vi "encoder2_test_v1.vi"() -> ()   [LabVIEW 2014]
uses:
  <vilib>/rvi/FXPMathLib/FxpSinAndCos/subVIs/nifxpmath_SinAndCos_SimConfig.ctl
  <vilib>/rvi/Emulation/niFpgaGetClockAttributes.vi
  <vilib>/rvi/Emulation/niFpgaSctlEmulationGetInTimedLoop.vi
  <vilib>/rvi/Emulation/niFpgaEmulationReportErrorSimple.vi
  <vilib>/rvi/eio/common/nirviEmuTemplateMethod_errors.vi
  <vilib>/rvi/Emulation/niFpgaProcessEmulError.vi
  <vilib>/rvi/Emulation/niFpgaCriticalErrorInLSC.vi
  <vilib>/rvi/interface/RandomDataEmulation/nirviRandomDataMultiElementFPGAFIFO.vi
  <instcachedir>/0/nirviRandomDataMultiElementFPGAFIFO_AD0CFC12EF974623A9C2E4184BC062B2.lvgen/nirviRandomDataMultiElementFPGAFIFO_AD0CFC12EF974623A9C2E4184BC062B2_028.vi
  <vilib>/rvi/interface/RandomDataEmulation/niFpgaRandomDataHandleErrors.vi
  <vilib>/rvi/FXPMathLib/FxpSinAndCos/simVIs/DllFxpSinAndCosTemp_sub.vi
  <vilib>/eio/EIONode/EIONode.xnode
  <vilib>/rvi/FXPMathLib/FxpMul/XNode/nifxpmath_Multiplier.xnode
  <vilib>/rvi/DataTransferAndStorage/Container/XNode/niFpgaContainer.xnode
  <vilib>/rvi/interface/RandomDataEmulation/nirviRandomDataFpgaMultiElementTemplate.vi
  <vilib>/rvi/FXPMathLib/FxpSinAndCos/XNode/nifxpmath_SinAndCos.xnode
  <vilib>/rvi/FXPMathLib/FxpSub/XNode/nifxpmath_Sub.xnode
  <vilib>/rvi/FXPMathLib/sim/FxpSim.dll
panel:
  in  "Tc_Mavg_mot (uSec)":i32 caption="D_d_M_avg_Tc (uSec)"
  out "omega_mot (M_avg)":fxp<+/-,40,19>
  out "D_d_mot (M_avg)":fxp<+/-,40,19>
  out "omega_mag 2":fxp<+/-,36,13>
  out "D_d_mag 2":fxp<+/-,36,16>
  in  "Tc_Mavg_mag  (uSec)":i32 caption="D_d_M_avg_Tc (uSec)"
  out "D_d_mag (M_avg)":fxp<+/-,40,19>
  out "omega_mag (M_avg)":fxp<+/-,40,19>
  in  "Velocity Est. (mag)":i16(ring) items=["T method", "Mavg method"]
  out "rad (NrTheta)":fxp<+/-,40,20>
  out "D (mm)":fxp<+/-,32,7>
  out "Dr_ramp2":fxp<+/-,64,21>
  out "Ts (s)":fxp<+/-,32,6>
  in  "Dr_ramp (mm)":fxp<+/-,33,7>
  out "Dr_ramp":fxp<+/-,64,21>
  in  "Vr (mm/s)":fxp<+/-,33,7>
  out "omega (rad/s)":fxp<+/-,36,13>
  in  "Encoder":i16(ring) items=["Motor", "Magnetic"]
  in  "Dr_step":fxp<+/-,33,7>
  out "Dr":fxp<+/-,33,10>
  in  "Command type":i16(ring) items=["Step", "Sine", "Ramp", "Ramp2"]
  out "Fmr_P":fxp<+/-,30,15>
  in  "Kp":fxp<+/-,27,14>
  out "D_error":fxp<+/-,36,11>
  out "Dr_sin_d":fxp<+/-,51,12>
  out "Sin omega":fxp<+,20,4>
  out "Dr_sin":fxp<+/-,33,10>
  in  "Sin Mag.":fxp<+/-,32,7>
  in  "Sine frequency (Hz)":fxp<+,16,5>=2.0
  out "Time now (s)":fxp<+,52,14>
  out "va":fxp<+/-,36,7>
  out "vb":fxp<+/-,37,8>
  out "vd_F":fxp<+/-,20,5>
  out "vq_F":fxp<+/-,20,5> format="%.57g"
  in  "Stop Motor":bool
  in  "Ini coe.":bool
  out "D_d_mag":fxp<+/-,36,13>
  out "omega_mag":fxp<+/-,36,13>
  out "D_mag":fxp<+/-,32,7>
  in  "Mag. factor":fxp<+/-,20,2>
  out "mt_mag.":u32
  out "D_d_mot":fxp<+/-,36,13>
  in  "Belt_screw":fxp<+/-,7,7>
  in  "Belt_motor":fxp<+/-,6,6>
  out "D_mot":fxp<+/-,32,7>
  out "rad_mag.":fxp<+/-,40,20>
  out "rad_mot":fxp<+/-,40,20>
  out "mt":u32
  out "omega_mot":fxp<+/-,36,13>
  in  "mt0":u32
  out "Mag. Encoder Position":i32
  in  "Encoder Reset":bool
  out "Encoder Position":i32
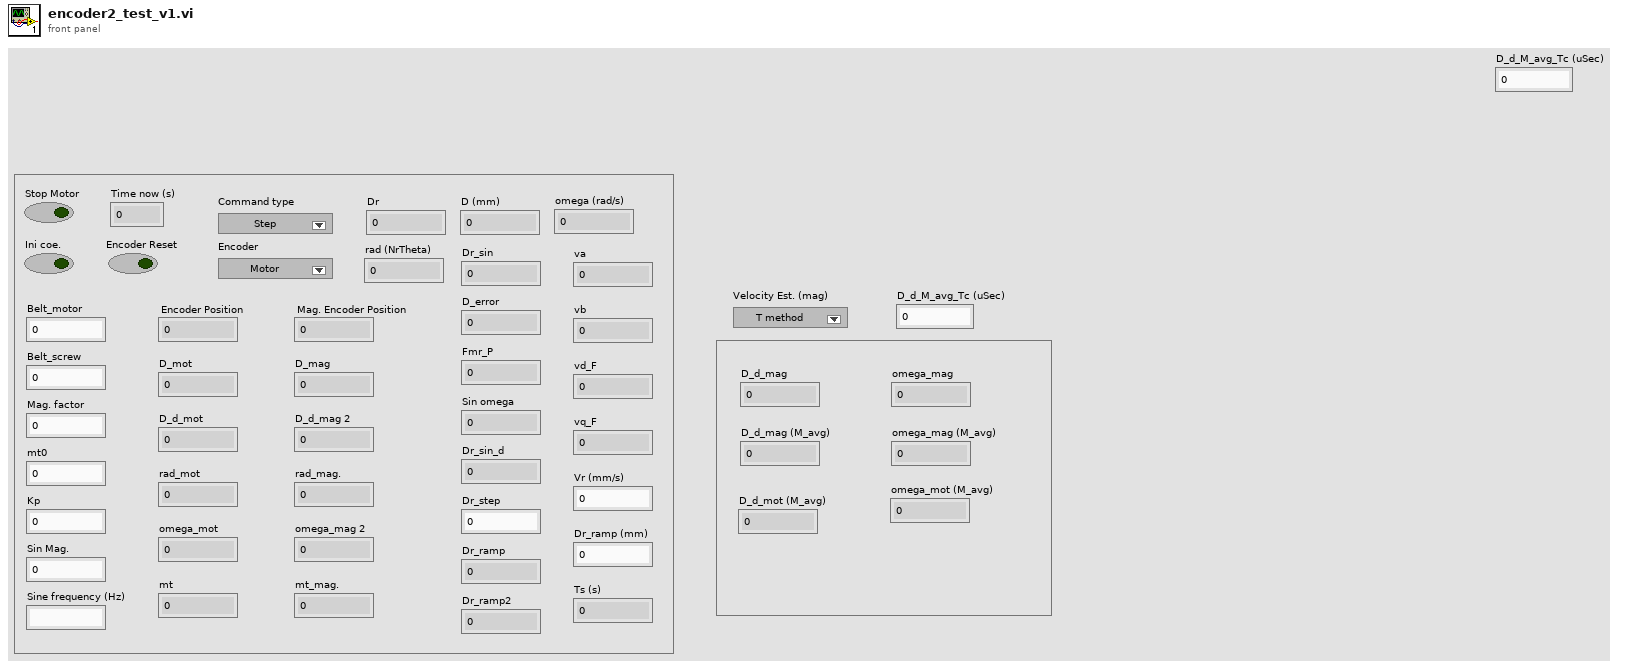
[diagram p1: front panel]
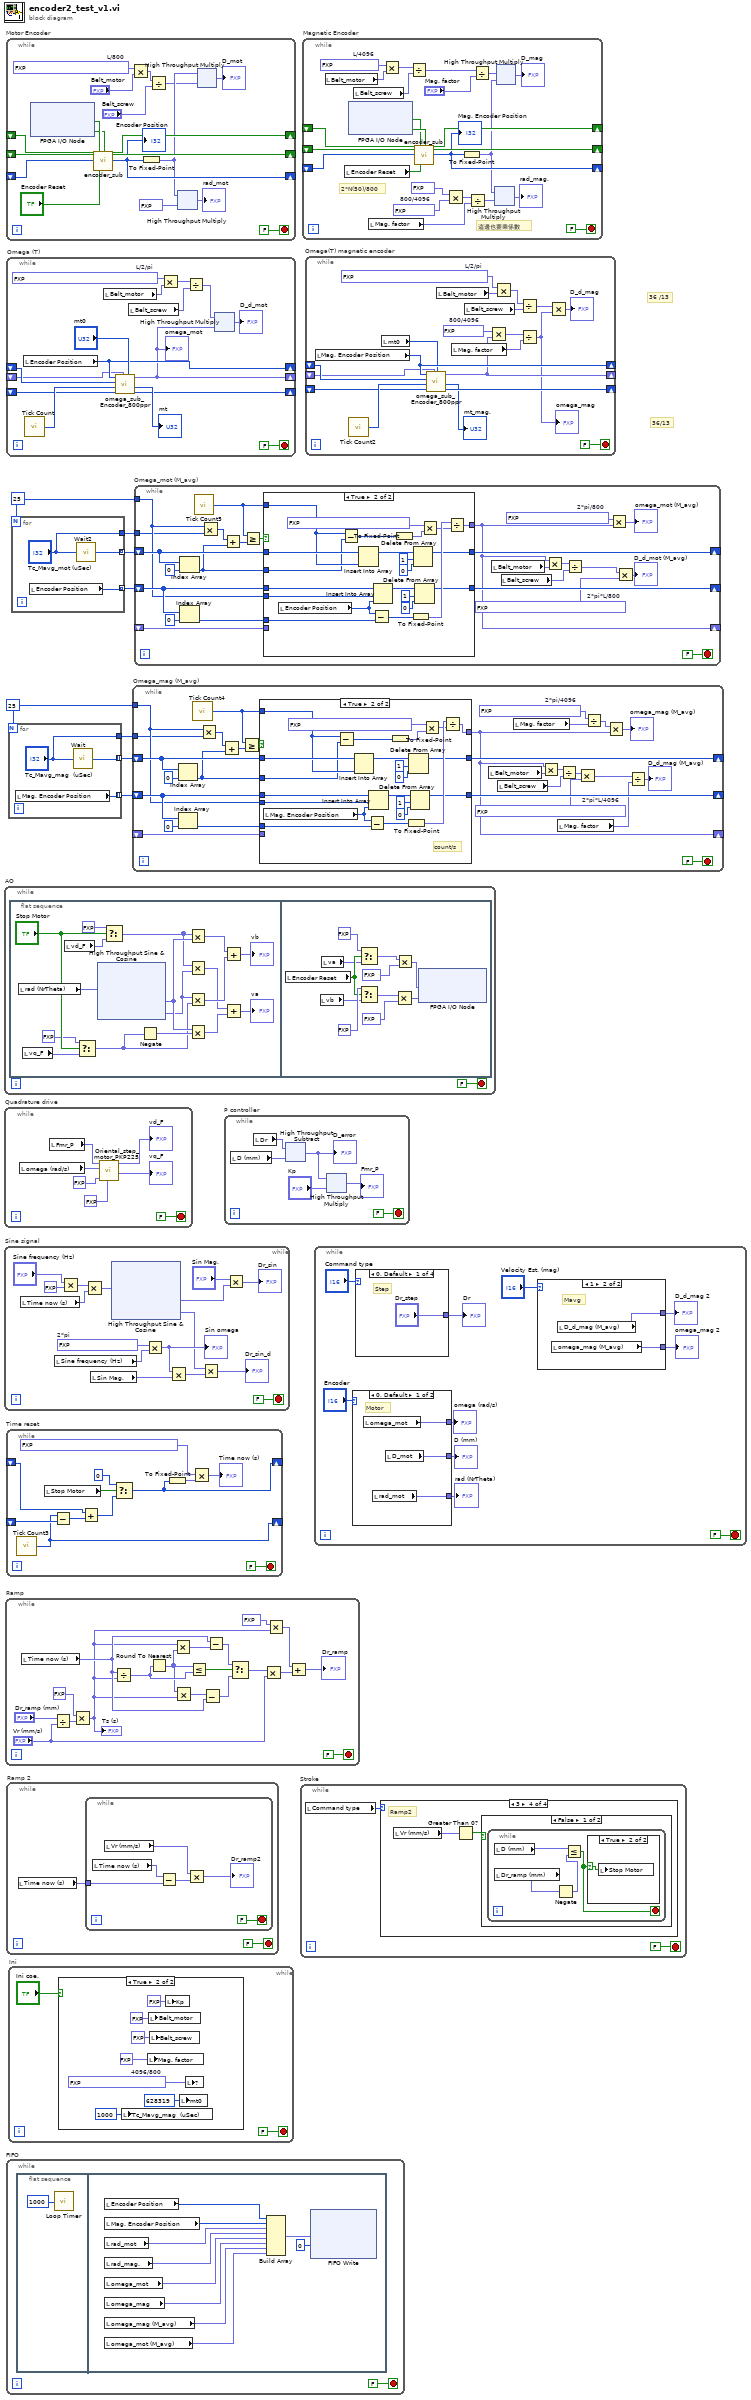
[diagram p0: block diagram]
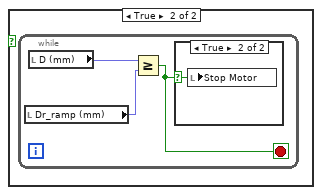
[diagram p8: hidden frame]
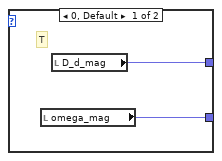
[diagram p10: hidden frame]
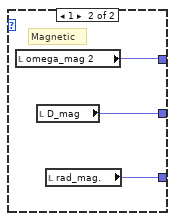
[diagram p11: hidden frame]
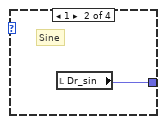
[diagram p12: hidden frame]
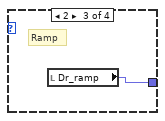
[diagram p13: hidden frame]
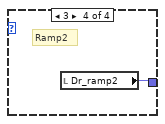
[diagram p14: hidden frame]
diagram:
  w4 = 25
  w8 = 25
  # "36/13"
  # "36 /13"
  n1 = while "AO" {
    stop <- FALSE stop-if-true
    n2 = flat-sequence {
      frame #0 {
        n3 = local read "rad (NrTheta)"() -> (w26:fxp<+/-,40,20>)
        n4 = local read "vq_F"() -> (w22:fxp<+/-,20,5>)
        n5 = local read "vd_F"() -> (w21:fxp<+/-,20,5>)
        n6 = Select(t=fxp<+,1,1> 0.0, s="Stop Motor", f=w22) -> (s? t:f=w12:fxp<+/-,20,5>)
        n7 = xnode "High Throughput Sine & Cosine"("x (pi)"=w26) -> ("sin(x)"=w16:fxp<+/-,16,2>, "cos(x)"=w14:fxp<+/-,16,2>)
        n8 = Select(t=fxp<+,1,1> 0.0, s="Stop Motor", f=w21) -> (s? t:f=w15:fxp<+/-,20,5>)
        n9 = Negate(x=w12) -> (-x=w13:fxp<+/-,21,6>)
        n10 = Multiply(x=w15, y=w16) -> (x*y=w20:fxp<+/-,36,7>)
        n11 = Multiply(x=w15, y=w14) -> (x*y=w18:fxp<+/-,36,7>)
        n12 = Multiply(x=w14, y=w12) -> (x*y=w19:fxp<+/-,36,7>)
        n13 = Multiply(x=w16, y=w13) -> (x*y=w17:fxp<+/-,35,6>)
        n14 = Add(x=w20, y=w19) -> (x+y=→"vb":fxp<+/-,37,8>)
        n15 = Add(x=w18, y=w17) -> (x+y=→"va":fxp<+/-,36,7>)
      }
      frame #1 {
        n16 = local read "Encoder Reset"() -> (w59:bool)
        n17 = local read "vb"() -> (w58:fxp<+/-,37,8>)
        n18 = local read "va"() -> (w57:fxp<+/-,36,7>)
        n19 = Select(t=fxp<+/-,20,5> 3.0 ("y"), s=w59, f=w57) -> (s? t:f=w64:fxp<+/-,36,7>)
        n20 = Select(t=fxp<+/-,20,5> 0.0 ("y"), s=w59, f=w58) -> (s? t:f=w65:fxp<+/-,37,8>)
        n21 = Multiply(x=w65, y=fxp<+/-,20,5> -0.5) -> (x*y=w62:fxp<+/-,55,11>)
        n22 = Multiply(x=w64, y=fxp<+/-,20,5> -0.5) -> (x*y=w61:fxp<+/-,55,11>)
        n23 = xnode "FPGA I/O Node"("Mod8/AO0"=w61, "Mod8/AO1"=w62) -> ()  [unwired: 2 in, 2 out]
      }
    }
  }
  n24 = while "Quadrature drive" {
    stop <- FALSE stop-if-true
    n25 = local read "omega (rad/s)"() -> (w68:fxp<+/-,36,13>)
    n26 = local read "Fmr_P"() -> (w70:fxp<+/-,30,15>)
    n27 = call "Oriental_step_motor_PKP225.vi"("F_Threshold"=fxp<+,12,12> 10.0, "dFmr"=fxp<+,1,1> 0.0 ("t"), "omega"=w68, "Fmr"=w70) -> ("vq_F"=→"vq_F":fxp<+/-,20,5>, "vd_F"=→"vd_F":fxp<+/-,20,5>)  [unwired: 6 in]
  }
  n28 = while "Sine signal" {
    stop <- FALSE stop-if-true
    w84 = fxp<+,20,3> 6.2831878662109375  # 2*pi
    n29 = local read "Time now (s)"() -> (w89:fxp<+,52,14>)
    n30 = local read "Sine frequency (Hz)"() -> (w83:fxp<+,16,5>)
    n31 = Multiply(x="Sine frequency (Hz)", y=fxp<+,1,2> 2.0 ("x")) -> (x*y=w90:fxp<+,16,6>)
    n32 = Multiply(x=w90, y=w89) -> (x*y=w88:fxp<+,64,20>)
    n33 = local read "Sin Mag."() -> (w82:fxp<+/-,32,7>)
    n34 = xnode "High Throughput Sine & Cosine"("x (pi)"=w88) -> ("sin(x)"=w86:fxp<+/-,16,2>, "cos(x)"=w79:fxp<+/-,16,2>)
    n35 = Multiply(x=w84, y=w83) -> (x*y=w81:fxp<+,36,8>)
    "Sin omega" <- w81
    n36 = Multiply(x=w81, y=w82) -> (x*y=w80:fxp<+/-,64,15>)
    n37 = Multiply(x=w79, y=w80) -> (x*y=→"Dr_sin_d":fxp<+/-,64,17>)
    n38 = Multiply(x="Sin Mag.", y=w86) -> (x*y=→"Dr_sin":fxp<+/-,48,9>)
  }
  n39 = while "Ramp" {
    stop <- FALSE stop-if-true
    n40 = local read "Time now (s)"() -> (w134:fxp<+,52,14>)
    n41 = Divide(x="Dr_ramp (mm)", y="Vr (mm/s)") -> (x/y=w123:fxp<+/-,64,34>)
    n42 = Multiply(x=fxp<+/-,3,3> 2.0, y=w123) -> (x*y=w121:fxp<+/-,64,37>)
    "Ts (s)" <- w121
    n43 = Divide(x=w134, y=w121) -> (x/y=w138:fxp<+/-,64,42>)
    n44 = Round To Nearest(number=w138) -> (nearest integer value=w137:fxp<+/-,43,43>)
    n45 = Multiply(x=w121, y=w137) -> (x*y=w136:fxp<+/-,64,79>)
    n46 = Multiply(x=w137, y=w121) -> (x*y=w135:fxp<+/-,64,79>)
    n47 = Less Or Equal?(x=w137, y=w138) -> (x <= y?=w133:bool)
    n48 = Subtract(x=w135, y=w134) -> (x-y=w131:fxp<+/-,64,80>)
    n49 = Subtract(x=w134, y=w136) -> (x-y=w132:fxp<+/-,64,80>)
    n50 = Select(t=w132, s=w133, f=w131) -> (s? t:f=w130:fxp<+/-,64,80>)
    n51 = Multiply(x=w130, y="Vr (mm/s)") -> (x*y=w127:fxp<+/-,64,87>)
    n52 = Multiply(x=fxp<+/-,2,1> -0.5, y=w121) -> (x*y=w126:fxp<+/-,64,38>)
    n53 = Add(x=w126, y=w127) -> (x+y=→"Dr_ramp":fxp<+/-,64,88>)
  }
  n54 = while "Motor Encoder" {
    shift-right: [w153] -> _
    shift-left: _ -> [w156]
    shift-right: [w152] -> _
    shift-left: _ -> [w157]
    shift-right: [w151] -> _
    shift-left: _ -> [w158]
    stop <- FALSE stop-if-true
    w142 = fxp<+/-,20,-5> 0.002499997615814209  # L/800
    n55 = xnode "FPGA I/O Node"() -> ("Mod4/DI0"=w155:bool, "Mod4/DI1"=w154:bool)  [unwired: 2 in, 2 out]
    n56 = call "encoder_sub.vi"("A_pre"=w156, "B_pre"=w157, "Encoder Position_pre"=w158, "A input"=w155, "Encoder Position Reset"="Encoder Reset", "B input"=w154) -> ("A"=w153:bool, "B"=w152:bool, "Encoder Position (Counts)"=w151:i32)  [unwired: 19 in]
    "Encoder Position" <- w151
    n57 = Multiply(x=w142, y="Belt_motor") -> (x*y=w144:fxp<+/-,26,1>)
    n58 = To Fixed-Point(number=w151) -> (fixed-point=w146:fxp<+/-,32,32>)  [unwired: 1 in]
    n59 = Divide(x=w144, y="Belt_screw") -> (x/y=w143:fxp<+/-,33,1>)
    n60 = xnode ("High Throughput Multiply")("x"=w146, "y"=fxp<+/-,16,1> 0.125) -> ("x*y"=→"rad_mot":fxp<+/-,48,33>)
    n61 = xnode ("High Throughput Multiply")("x"=w146, "y"=w143) -> ("x*y"=→"D_mot":fxp<+/-,64,33>)
  }
  n62 = while "Time reset" {
    shift-right: [w162] -> _
    shift-left: _ -> [w167]
    shift-right: [w165] -> _
    shift-left: _ -> [w166]
    stop <- FALSE stop-if-true
    n63 = call "Tick Count3"() -> ("Tick Count(uSec)"=w165:u32)
    n64 = local read "Stop Motor"() -> (w170:bool)
    n65 = Subtract(x=w165, y=w166) -> (x-y=w169:u32)
    n66 = Add(x=w167, y=w169) -> (x+y=w168:u32)
    n67 = Select(t=u32 0, s=w170, f=w168) -> (s? t:f=w162:u32)
    n68 = To Fixed-Point(number=w162) -> (fixed-point=w164:fxp<+,32,32>)  [unwired: 1 in]
    n69 = Multiply(x=fxp<+,20,-18> 1.0000003385357559e-06, y=w164) -> (x*y=→"Time now (s)":fxp<+,52,14>)
  }
  n70 = while "FIFO" {
    stop <- FALSE stop-if-true
    n71 = flat-sequence {
      frame #0 {
        n72 = call "Loop Timer"("Count(uSec)"=u32 1000) -> ()  [unwired: 1 out]
      }
      frame #1 {
        n73 = local read "Encoder Position"() -> (w182:i32)
        n74 = local read "Mag. Encoder Position"() -> (w181:i32)
        n75 = local read "rad_mot"() -> (w180:fxp<+/-,40,20>)
        n76 = local read "rad_mag."() -> (w179:fxp<+/-,40,20>)
        n77 = local read "omega_mot"() -> (w178:fxp<+/-,36,13>)
        n78 = local read "omega_mag"() -> (w177:fxp<+/-,36,13>)
        n79 = local read "omega_mag (M_avg)"() -> (w176:fxp<+/-,40,19>)
        n80 = local read "omega_mot (M_avg)"() -> (w173:fxp<+/-,40,19>)
        n81 = Build Array(w182, w181, w180, w179, w178, w177, w176, w173) -> (w174:fxp<+/-,55,32>[])
        n82 = xnode ("FIFO Write")("Element"=w174, "Timeout"=0) -> ()  [unwired: 1 in, 2 out]
      }
    }
  }
  n83 = while "Omega (T)" {
    shift-right: [w196] -> _
    shift-left: _ -> [w197]
    shift-right: [w185] -> _
    shift-left: _ -> [w193]
    shift-right: [w194] -> _
    shift-left: _ -> [w191]
    stop <- FALSE stop-if-true
    w190 = fxp<+/-,32,0> 0.3183098859153688  # L/2/pi
    n84 = local read "Encoder Position"() -> (w196:i32)
    n85 = call "Tick Count"() -> ("Tick Count(Ticks)"=w192:u32)
    n86 = local read "Belt_motor"() -> (w189:fxp<+/-,6,6>)
    n87 = call "omega_sub_Encoder_800ppr.vi"("mt0"="mt0", "omega_pre"=w193, "ticks_m_pre"=w191, "ticks"=w192, "count_pre"=w197, "count"=w196) -> ("ticks_m"=w194:u32, "mt"=→"mt":u32, "omega"=w185:fxp<+/-,36,13>)  [unwired: 3 in]
    "omega_mot" <- w185
    n88 = local read "Belt_screw"() -> (w187:fxp<+/-,7,7>)
    n89 = Multiply(x=w190, y=w189) -> (x*y=w188:fxp<+/-,38,6>)
    n90 = Divide(x=w188, y=w187) -> (x/y=w186:fxp<+/-,45,6>)
    n91 = xnode ("High Throughput Multiply")("x"=w186, "y"=w185) -> ("x*y"=→"D_d_mot":fxp<+/-,64,19>)
  }
  n92 = while "Ramp 2" {
    stop <- FALSE stop-if-true
    n93 = local read "Time now (s)"() -> (w200:fxp<+,52,14>)
    n94 = while {
      tunnel: w200 -> [w205]
      stop <- FALSE stop-if-true
      n95 = local read "Time now (s)"() -> (w206:fxp<+,52,14>)
      n96 = local read "Vr (mm/s)"() -> (w203:fxp<+/-,33,7>)
      n97 = Subtract(x=w206, y=w205) -> (x-y=w204:fxp<+/-,53,15>)
      n98 = Multiply(x=w203, y=w204) -> (x*y=→"Dr_ramp2":fxp<+/-,64,21>)
    }
  }
  n99 = for {
    N: w8 -> [_]
    tunnel: ["Tc_Mavg_mag  (uSec)"] -> w5
    tunnel: [w208] -> w7 mode=indexing
    tunnel: [w207] -> w6 mode=indexing
    n100 = local read "Mag. Encoder Position"() -> (w207:i32)
    n101 = call "Wait"("Count(uSec)"="Tc_Mavg_mag  (uSec)") -> ("Tick Count(uSec)"=w208:u32)
  }
  n102 = while "Ini" {
    stop <- FALSE stop-if-true
    n103 = case shown="True" "Ini coe." {
      frame False {
      }
      frame True {
        w212 = fxp<+/-,36,14> 5.119999885559082  # 4096/800
        n104 = local write "Tc_Mavg_mag  (uSec)"(u32 1000 ("D_d_M_avg_Tc (uSec)")) -> ()
        n105 = local write "Mag. factor"(fxp<+/-,20,2> 1.0 ("Coorection factor")) -> ()
        n106 = local write "Belt_motor"(fxp<+/-,6,6> 14.0 ("Belt_motor")) -> ()
        n107 = local write "Belt_screw"(fxp<+/-,7,7> 36.0 ("Belt_screw")) -> ()
        n108 = local write "Kp"(fxp<+/-,27,14> 50.0 ("Kp")) -> ()
        n109 = local write "mt0"(u32 628319 ("mt0")) -> ()
        n110 = local write item#-1(w212) -> ()
      }
    }
  }
  n111 = for {
    N: w4 -> [_]
    tunnel: ["Tc_Mavg_mot (uSec)"] -> w2
    tunnel: [w220] -> w3 mode=indexing
    tunnel: [w219] -> w1 mode=indexing
    n112 = local read "Encoder Position"() -> (w219:i32)
    n113 = call "Wait2"("Count(uSec)"="Tc_Mavg_mot (uSec)") -> ("Tick Count(uSec)"=w220:u32)
  }
  n114 = while "Omega_mag (M_avg)" {
    tunnel: w8 -> [w243]
    shift-right: [w236] -> _
    shift-left: w7 -> [w247]
    shift-right: [w222] -> _
    shift-left: _ -> [w238]
    shift-right: [w237] -> _
    shift-left: w6 -> [w246]
    tunnel: w5 -> [w240]
    stop <- FALSE stop-if-true
    w227 = fxp<+/-,27,3> 0.0015339851379394531  # 2*pi/4096
    w230 = fxp<+/-,32,0> 0.003067961661145091  # 2*pi*L/4096
    n115 = Index Array(array=w247, index=0) -> (element=w241:u32)
    n116 = Index Array(array=w246, index=0) -> (element=w242:i32)
    n117 = call "Tick Count4"() -> ("Tick Count(uSec)"=w244:u32)
    n118 = Multiply(x=w243, y=w240) -> (x*y=w248:i32)
    n119 = Add(x=w248, y=w241) -> (x+y=w245:u32)
    n120 = Greater Or Equal?(x=w244, y=w245) -> (x >= y?=w239:bool)
    n121 = case shown="True" w239 {
      tunnel: w247 -> [w253 w270]
      tunnel: w246 -> [w252 w269]
      tunnel: w244 -> [_ w265]
      tunnel: w243 -> [_ w268]
      tunnel: w242 -> [_ w266]
      tunnel: w241 -> [_ w264]
      tunnel: w238 -> [w251 _]
      tunnel: [w252 w260] -> w237
      tunnel: [w253 w259] -> w236
      tunnel: [w251 w258] -> w222
      frame False {
      }
      frame True {
        # "count/s"
        n122 = local read "Mag. Encoder Position"() -> (w267:i32)
        n123 = Subtract(x=w265, y=w264) -> (x-y=w262:u32)
        n124 = Insert Into Array(array=w270, new element=w265) -> (w271:u32[])  [unwired: 1 in]
        n125 = Subtract(x=w267, y=w266) -> (x-y=w257:i32)
        n126 = Insert Into Array(array=w269, index=w268, new element=w267) -> (w272:i32[])
        n127 = To Fixed-Point(number=w262) -> (fixed-point=w254:fxp<+,32,32>)  [unwired: 1 in]
        n128 = To Fixed-Point(number=w257) -> (fixed-point=w261:fxp<+/-,32,32>)  [unwired: 1 in]
        n129 = Delete From Array(array=w271, length=1, index=0) -> (array with subset deleted=w259:u32[])  [unwired: 1 out]
        n130 = Delete From Array(array=w272, length=1, index=0) -> (array with subset deleted=w260:i32[])  [unwired: 1 out]
        n131 = Multiply(x=fxp<+/-,15,-15> 1.000240445137024e-06, y=w254) -> (x*y=w256:fxp<+/-,47,17>)
        n132 = Divide(x=w261, y=w256) -> (x/y=w258:fxp<+/-,64,32>)
      }
    }
    n133 = local read "Belt_motor"() -> (w234:fxp<+/-,6,6>)
    n134 = local read "Belt_screw"() -> (w233:fxp<+/-,7,7>)
    n135 = local read "Mag. factor"() -> (w228:fxp<+/-,20,2>)
    n136 = Multiply(x=w222, y=w234) -> (x*y=w235:fxp<+/-,64,38>)
    n137 = local read "Mag. factor"() -> (w224:fxp<+/-,20,2>)
    n138 = Divide(x=w235, y=w233) -> (x/y=w229:fxp<+/-,64,39>)
    n139 = Multiply(x=w229, y=w230) -> (x*y=w225:fxp<+/-,64,39>)
    n140 = Divide(x=w227, y=w228) -> (x/y=w226:fxp<+/-,48,22>)
    n141 = Multiply(x=w226, y=w222) -> (x*y=→"omega_mag (M_avg)":fxp<+/-,64,53>)
    n142 = Divide(x=w225, y=w224) -> (x/y=→"D_d_mag (M_avg)":fxp<+/-,64,58>)
  }
  n143 = while "Omega_mot (M_avg)" {
    tunnel: w4 -> [w293]
    shift-right: [w286] -> _
    shift-left: w3 -> [w297]
    shift-right: [w278] -> _
    shift-left: _ -> [w288]
    shift-right: [w287] -> _
    shift-left: w1 -> [w296]
    tunnel: w2 -> [w290]
    stop <- FALSE stop-if-true
    w281 = fxp<+/-,32,0> 0.015707963379099965  # 2*pi*L/800
    w279 = fxp<+/-,27,3> 0.007853984832763672  # 2*pi/800
    n144 = Index Array(array=w297, index=0) -> (element=w291:u32)
    n145 = Index Array(array=w296, index=0) -> (element=w292:i32)
    n146 = call "Tick Count5"() -> ("Tick Count(uSec)"=w294:u32)
    n147 = Multiply(x=w293, y=w290) -> (x*y=w298:i32)
    n148 = Add(x=w298, y=w291) -> (x+y=w295:u32)
    n149 = Greater Or Equal?(x=w294, y=w295) -> (x >= y?=w289:bool)
    n150 = case shown="True" w289 {
      tunnel: w297 -> [w303 w320]
      tunnel: w296 -> [w302 w319]
      tunnel: w294 -> [_ w315]
      tunnel: w293 -> [_ w318]
      tunnel: w292 -> [_ w316]
      tunnel: w291 -> [_ w314]
      tunnel: w288 -> [w301 _]
      tunnel: [w302 w310] -> w287
      tunnel: [w303 w309] -> w286
      tunnel: [w301 w308] -> w278
      frame False {
      }
      frame True {
        n151 = local read "Encoder Position"() -> (w317:i32)
        n152 = Subtract(x=w315, y=w314) -> (x-y=w312:u32)
        n153 = Insert Into Array(array=w320, new element=w315) -> (w321:u32[])  [unwired: 1 in]
        n154 = Subtract(x=w317, y=w316) -> (x-y=w307:i32)
        n155 = Insert Into Array(array=w319, index=w318, new element=w317) -> (w322:i32[])
        n156 = To Fixed-Point(number=w312) -> (fixed-point=w305:fxp<+,32,32>)  [unwired: 1 in]
        n157 = To Fixed-Point(number=w307) -> (fixed-point=w311:fxp<+/-,32,32>)  [unwired: 1 in]
        n158 = Delete From Array(array=w321, length=1, index=0) -> (array with subset deleted=w309:u32[])  [unwired: 1 out]
        n159 = Delete From Array(array=w322, length=1, index=0) -> (array with subset deleted=w310:i32[])  [unwired: 1 out]
        n160 = Multiply(x=fxp<+/-,15,-15> 1.000240445137024e-06, y=w305) -> (x*y=w306:fxp<+/-,47,17>)
        n161 = Divide(x=w311, y=w306) -> (x/y=w308:fxp<+/-,64,32>)
      }
    }
    n162 = local read "Belt_motor"() -> (w284:fxp<+/-,6,6>)
    n163 = local read "Belt_screw"() -> (w283:fxp<+/-,7,7>)
    n164 = Multiply(x=w278, y=w284) -> (x*y=w285:fxp<+/-,64,38>)
    n165 = Divide(x=w285, y=w283) -> (x/y=w277:fxp<+/-,64,39>)
    n166 = Multiply(x=w279, y=w278) -> (x*y=→"omega_mot (M_avg)":fxp<+/-,64,35>)
    n167 = Multiply(x=w277, y=w281) -> (x*y=→"D_d_mot (M_avg)":fxp<+/-,64,39>)
  }
  n168 = while "P controller" {
    stop <- FALSE stop-if-true
    n169 = local read "D (mm)"() -> (w331:fxp<+/-,32,7>)
    n170 = local read "Dr"() -> (w326:fxp<+/-,33,10>)
    n171 = xnode "High Throughput Subtract"("x"=w326, "y"=w331) -> ("x-y"=w330:fxp<+/-,36,11>)
    "D_error" <- w330
    n172 = xnode ("High Throughput Multiply")("x"=w330, "y"="Kp") -> ("x*y"=→"Fmr_P":fxp<+/-,63,25>)
  }
  n173 = while "Stroke" {
    stop <- FALSE stop-if-true
    n174 = local read "Command type"() -> (w333:i16)
    n175 = case shown="3" w333 {
      frame 0, Default {
        # "Step"
      }
      frame 1 {
        # "Sine"
      }
      frame 2 {
        # "Ramp"
      }
      frame 3 {
        # "Ramp2"
        n176 = local read "Vr (mm/s)"() -> (w335:fxp<+/-,33,7>)
        n177 = Greater Than 0?(x=w335) -> (x > 0?=w334:bool)
        n178 = case shown="False" w334 {
          frame False {
            n179 = while {
              stop <- w338 stop-if-true
              n180 = local read "D (mm)"() -> (w339:fxp<+/-,32,7>)
              n181 = local read "Dr_ramp (mm)"() -> (w337:fxp<+/-,33,7>)
              n182 = Negate(x=w337) -> (-x=w336:fxp<+/-,34,8>)
              n183 = Less Or Equal?(x=w339, y=w336) -> (x <= y?=w338:bool)
              n184 = case shown="True" w338 {
                selector: w338 -> [_ w340]
                frame False {
                }
                frame True {
                  n185 = local write "Stop Motor"(w340) -> ()
                }
              }
            }
          }
          frame True {
            n186 = while {
              stop <- w341 stop-if-true
              n187 = local read "Dr_ramp (mm)"() -> (w342:fxp<+/-,33,7>)
              n188 = local read "D (mm)"() -> (w343:fxp<+/-,32,7>)
              n189 = Greater Or Equal?(x=w343, y=w342) -> (x >= y?=w341:bool)
              n190 = case shown="True" w341 {
                selector: w341 -> [_ w344]
                frame False {
                }
                frame True {
                  n191 = local write "Stop Motor"(w344) -> ()
                }
              }
            }
          }
        }
      }
    }
  }
  n192 = while "Magnetic Encoder" {
    shift-right: [w365] -> _
    shift-left: _ -> [w366]
    shift-right: [w368] -> _
    shift-left: _ -> [w369]
    shift-right: [w362] -> _
    shift-left: _ -> [w367]
    stop <- FALSE stop-if-true
    w349 = fxp<+,20,0> 0.1953125  # 800/4096
    w359 = fxp<+/-,20,-5> 0.00048828125  # L/4096
    # "2*N(50)/800"
    # "這邊也要乘係數"
    n193 = local read "Belt_motor"() -> (w358:fxp<+/-,6,6>)
    n194 = local read "Encoder Reset"() -> (w351:bool)
    n195 = xnode "FPGA I/O Node"() -> ("Mod4/DI3"=w363:bool, "Mod4/DI4"=w364:bool)  [unwired: 2 in, 2 out]
    n196 = local read "Belt_screw"() -> (w356:fxp<+/-,7,7>)
    n197 = local read "Mag. factor"() -> (w345:fxp<+/-,20,2>)
    n198 = Multiply(x=w359, y=w358) -> (x*y=w357:fxp<+/-,26,1>)
    n199 = Divide(x=w357, y=w356) -> (x/y=w353:fxp<+/-,33,1>)
    n200 = call "encoder_sub.vi"("A_pre"=w366, "B_pre"=w369, "Encoder Position_pre"=w367, "A input"=w363, "Encoder Position Reset"=w351, "B input"=w364) -> ("A"=w365:bool, "B"=w368:bool, "Encoder Position (Counts)"=w362:i32)  [unwired: 19 in]
    "Mag. Encoder Position" <- w362
    n201 = Multiply(x=fxp<+/-,16,1> 0.125 ("y"), y=w349) -> (x*y=w346:fxp<+/-,36,1>)
    n202 = To Fixed-Point(number=w362) -> (fixed-point=w355:fxp<+/-,32,32>)  [unwired: 1 in]
    n203 = Divide(x=w346, y=w345) -> (x/y=w348:fxp<+/-,56,19>)
    n204 = Divide(x=w353, y="Mag. factor") -> (x/y=w354:fxp<+/-,53,19>)
    n205 = xnode ("High Throughput Multiply")("x"=w355, "y"=w348) -> ("x*y"=→"rad_mag.":fxp<+/-,64,51>)
    n206 = xnode ("High Throughput Multiply")("x"=w354, "y"=w355) -> ("x*y"=→"D_mag":fxp<+/-,64,51>)
  }
  n207 = while "Omega(T) magnetic encoder" {
    shift-right: [w384] -> _
    shift-left: _ -> [w383]
    shift-right: [w376] -> _
    shift-left: _ -> [w377]
    shift-right: [w380] -> _
    shift-left: _ -> [w381]
    stop <- FALSE stop-if-true
    w375 = fxp<+,20,0> 0.1953125  # 800/4096
    w387 = fxp<+/-,32,0> 0.3183098859153688  # L/2/pi
    n208 = local read "Mag. Encoder Position"() -> (w384:i32)
    n209 = call "Tick Count2"() -> ("Tick Count(Ticks)"=w382:u32)
    n210 = local read "mt0"() -> (w378:u32)
    n211 = call "omega_sub_Encoder_800ppr.vi"("mt0"=w378, "omega_pre"=w377, "ticks_m_pre"=w381, "ticks"=w382, "count_pre"=w383, "count"=w384) -> ("ticks_m"=w380:u32, "mt"=→"mt_mag.":u32, "omega"=w376:fxp<+/-,36,13>)  [unwired: 3 in]
    n212 = local read "Belt_motor"() -> (w386:fxp<+/-,6,6>)
    n213 = local read "Mag. factor"() -> (w370:fxp<+/-,20,2>)
    n214 = local read "Belt_screw"() -> (w385:fxp<+/-,7,7>)
    n215 = Multiply(x=w375, y=w376) -> (x*y=w371:fxp<+/-,40,14>)
    n216 = Multiply(x=w387, y=w386) -> (x*y=w388:fxp<+/-,38,6>)
    n217 = Divide(x=w388, y=w385) -> (x/y=w374:fxp<+/-,32,6>)
    n218 = Divide(x=w371, y=w370) -> (x/y=w373:fxp<+/-,61,33>)
    "omega_mag" <- w373
    n219 = Multiply(x=w374, y=w373) -> (x*y=→"D_d_mag":fxp<+/-,36,11>)
  }
  n220 = while {
    stop <- FALSE stop-if-true
    n221 = case shown="0, Default" "Encoder" {
      tunnel: [w406 w409] -> w396
      tunnel: [w405 w408] -> w395
      tunnel: [w404 w407] -> w394
      frame 0, Default {
        # "Motor"
        n222 = local read "omega_mot"() -> (w406:fxp<+/-,36,13>)
        n223 = local read "rad_mot"() -> (w404:fxp<+/-,40,20>)
        n224 = local read "D_mot"() -> (w405:fxp<+/-,32,7>)
      }
      frame 1 {
        # "Magnetic"
        n225 = local read "omega_mag 2"() -> (w409:fxp<+/-,36,13>)
        n226 = local read "D_mag"() -> (w408:fxp<+/-,32,7>)
        n227 = local read "rad_mag."() -> (w407:fxp<+/-,40,20>)
      }
    }
    "omega (rad/s)" <- w396
    "D (mm)" <- w395
    "rad (NrTheta)" <- w394
    n228 = case shown="0, Default" "Command type" {
      tunnel: ["Dr_step" w411 w412 w413] -> w398
      frame 0, Default {
        # "Step"
      }
      frame 1 {
        # "Sine"
        n229 = local read "Dr_sin"() -> (w411:fxp<+/-,33,10>)
      }
      frame 2 {
        # "Ramp"
        n230 = local read "Dr_ramp"() -> (w412:fxp<+/-,64,21>)
      }
      frame 3 {
        # "Ramp2"
        n231 = local read "Dr_ramp2"() -> (w413:fxp<+/-,64,21>)
      }
    }
    "Dr" <- w398
    n232 = case shown="1" "Velocity Est. (mag)" {
      tunnel: [w401 w403] -> w392
      tunnel: [w400 w402] -> w391
      frame 0, Default {
        # "T"
        n233 = local read "omega_mag"() -> (w400:fxp<+/-,36,13>)
        n234 = local read "D_d_mag"() -> (w401:fxp<+/-,36,13>)
      }
      frame 1 {
        # "Mavg"
        n235 = local read "omega_mag (M_avg)"() -> (w402:fxp<+/-,40,19>)
        n236 = local read "D_d_mag (M_avg)"() -> (w403:fxp<+/-,40,19>)
      }
    }
    "D_d_mag 2" <- w392
    "omega_mag 2" <- w391
  }
